vi "FTW-Actor-GetNextJob.vi"(0 "FTW Actor Instance":refnum<class "FTW-Actor-Instance.lvclass">, 7 "Jobs Performed":i32, 11 "error in":errorcluster) -> (4 "FTW Actor Instance out":refnum<class "FTW-Actor-Instance.lvclass">, 6 "Event Structure Timeout":i32=20 format="%d msec", 8 "Job Name":string, 15 "error out":errorcluster)   [LabVIEW 2015, in "FTW-Actor-Instance.lvclass"]
uses:
  FTW-Actor-Instance.lvclass
  scheduler/FTW-Scheduler.lvclass
panel:
  # "Inputs"
  # "Outputs"
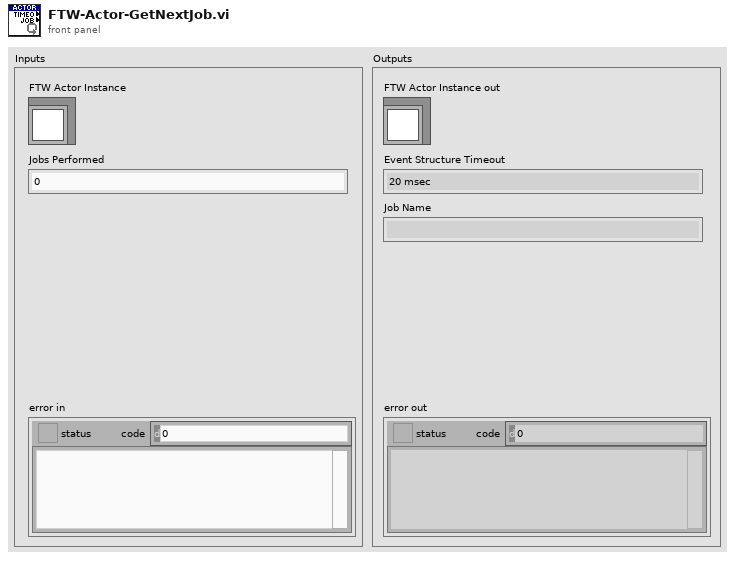
[diagram p1: front panel]
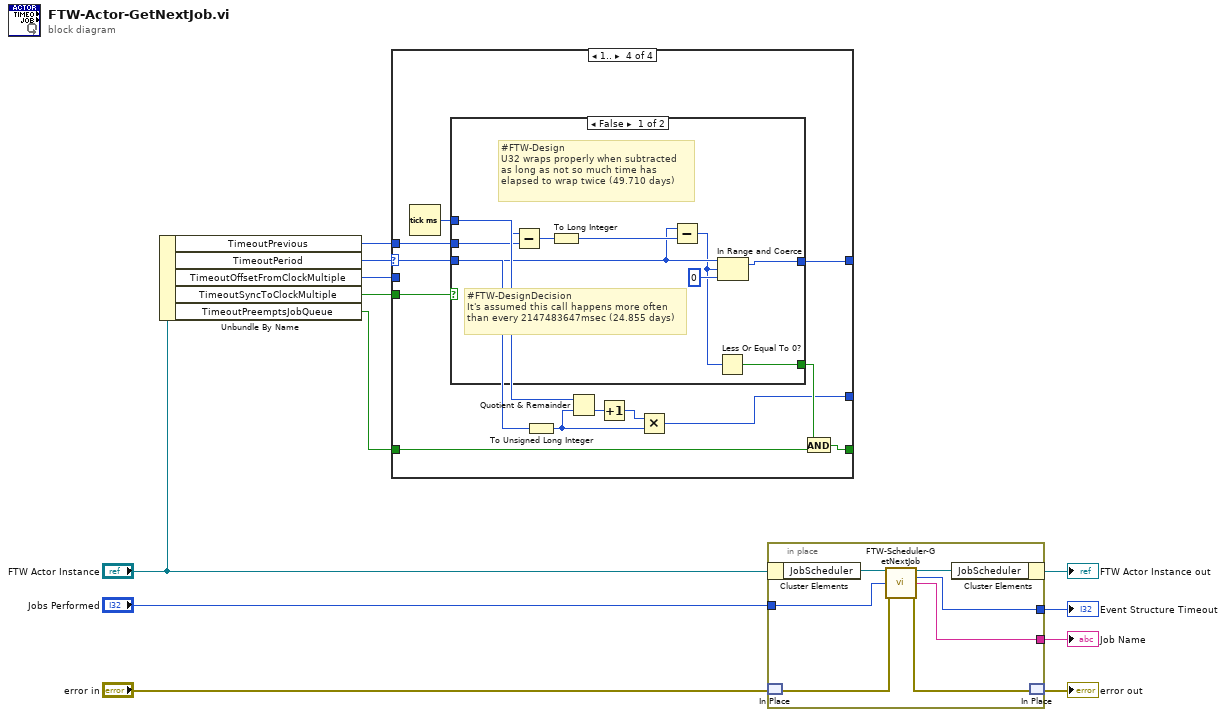
[diagram p0: block diagram]
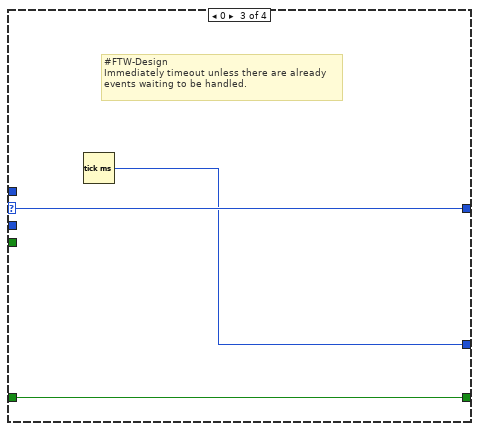
[diagram p4: hidden frame]
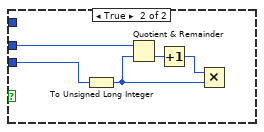
[diagram p5: hidden frame]
diagram:
  n1 = Unbundle By Name("FTW Actor Instance") -> ("TimeoutPrevious"=w8:u32, "TimeoutPeriod"=w9:i32, "TimeoutOffsetFromClockMultiple"=w6:i32, "TimeoutSyncToClockMultiple"=w4:bool, "TimeoutPreemptsJobQueue"=w5:bool)
  n2 = case shown="1.." w9 {
    selector: w9 -> [w13 w14 w17 w25]
    tunnel: w8 -> [_ _ _ w30]
    tunnel: [w13 w14 w17 w29] -> _
    tunnel: w6 -> [_ _ _ w22]
    tunnel: [_ _ w16 w20] -> _
    tunnel: w5 -> [_ _ w16 w21]
    tunnel: [_ _ w15 w19] -> _
    tunnel: w4 -> [_ _ _ w18]
    frame ..-2 {
      # "#FTW-Design\nThe Event Structure does not well-define\nbehavior for values below -1, so we'll pass\nthe value unchanged to allow it to choose\nits own semantics. Currently, behavior is\nthe same as if the value were -1."
    }
    frame -1 {
      # "#FTW-Design\nDo not timeout. The actor is intended to be\nentirely reactive and not proactive."
    }
    frame 0 {
      # "#FTW-Design\nImmediately timeout unless there are already\nevents waiting to be handled."
      n3 = Tick Count (ms)() -> (millisecond timer value=w15:u32)
    }
    frame 1.. {
      n4 = Tick Count (ms)() -> (millisecond timer value=w26:u32)
      n5 = case shown="False" w18 {
        tunnel: w30 -> [w39 w40]
        tunnel: [w35 _] -> w29
        tunnel: w26 -> [w34 _]
        tunnel: w25 -> [w33 w41]
        tunnel: [w31 _] -> w23
        frame False {
          # "#FTW-DesignDecision\nIt's assumed this call happens more often\nthan every 2147483647msec (24.855 days)"
          # "#FTW-Design\nU32 wraps properly when subtracted\nas long as not so much time has\nelapsed to wrap twice (49.710 days)"
          n6 = Subtract(x=w34, y=w39) -> (x-y=w37:u32)
          n7 = To Long Integer(number=w37) -> (32bit integer=w36:i32)
          n8 = Subtract(x=w33, y=w36) -> (x-y=w32:i32)
          n9 = Less Or Equal To 0?(x=w32) -> (x <= 0?=w31:bool)
          n10 = In Range and Coerce(upper limit=w33, x=w32, lower limit=0) -> (coerced(x)=w35:i32)  [unwired: 1 out]
        }
        frame True {
          n11 = To Unsigned Long Integer(number=w41) -> (unsigned 32bit integer=w44:u32)
          n12 = Quotient & Remainder(x=w40, y=w44) -> (floor(x/y)=w43:u32)  [unwired: 1 out]
          n13 = Increment(x=w43) -> (x+1=w42:u32)
          n14 = Multiply(x=w42, y=w44) -> ()  [unwired: 1 out]
        }
      }
      n15 = To Unsigned Long Integer(number=w25) -> (unsigned 32bit integer=w24:u32)
      n16 = Quotient & Remainder(x=w26, y=w24) -> (floor(x/y)=w27:u32)  [unwired: 1 out]
      n17 = Increment(x=w27) -> (x+1=w28:u32)
      n18 = Multiply(x=w28, y=w24) -> (x*y=w19:u32)
      n19 = And(x=w23, y=w21) -> (x .and. y?=w20:bool)
    }
  }
  n20 = in-place {
    in-place-border: [w49] -> w11
    in-place-border: "Jobs Performed" -> [w48]
    in-place-border: [w45] -> w3
    n21 = in-place-cluster #1("FTW Actor Instance") -> ("JobScheduler"=w51:refnum<class "FTW-Scheduler.lvclass">)
    n22 = in-place-match #2("error in") -> (w46:errorcluster)
    n23 = call "FTW-Scheduler-GetNextJob.vi"("FTW Job Scheduler"=w51, "Jobs Performed"=w48, "error in"=w46) -> ("FTW Job Scheduler out"=w50:refnum<class "FTW-Scheduler.lvclass">, "Time til Next Scheduled Job"=w45:i32, "Current Job"=w49:string, "error out"=w47:errorcluster)  [unwired: 9 in]
    n24 = in-place-cluster #1("JobScheduler"=w50) -> (→"FTW Actor Instance out":refnum<class "FTW-Actor-Instance.lvclass">)
    n25 = in-place-match #2(w47) -> (→"error out":errorcluster)
  }
  "Job Name" <- w11
  "Event Structure Timeout" <- w3
